vi "Periodic Tasks.vi"(8 "error in":errorcluster) -> ()   [LabVIEW 2020]
doc: "This VI runs in parallel to other robot code. It can contain as many user-defined periodic loops as you need. These can carry out PID or other sorts of timed response."
uses:
  <vilib>/Rock Robotics/WPI/Utilities/WPI_GetSetVariantRefNum.vi
  Robot Global Data.vi
  <vilib>/Rock Robotics/Network Tables/NT Write Number.vi
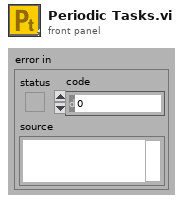
[diagram p1: front panel]
types:
  T1 = typedef "WPI_JoystickDevRef.ctl" = cluster{"Device":T2}
  T2 = typedef "WPI_JoystickDeviceEnum.ctl" = enum16{"USB 0", "USB 1", "USB 2", "USB 3", "USB 4", "USB 5"}
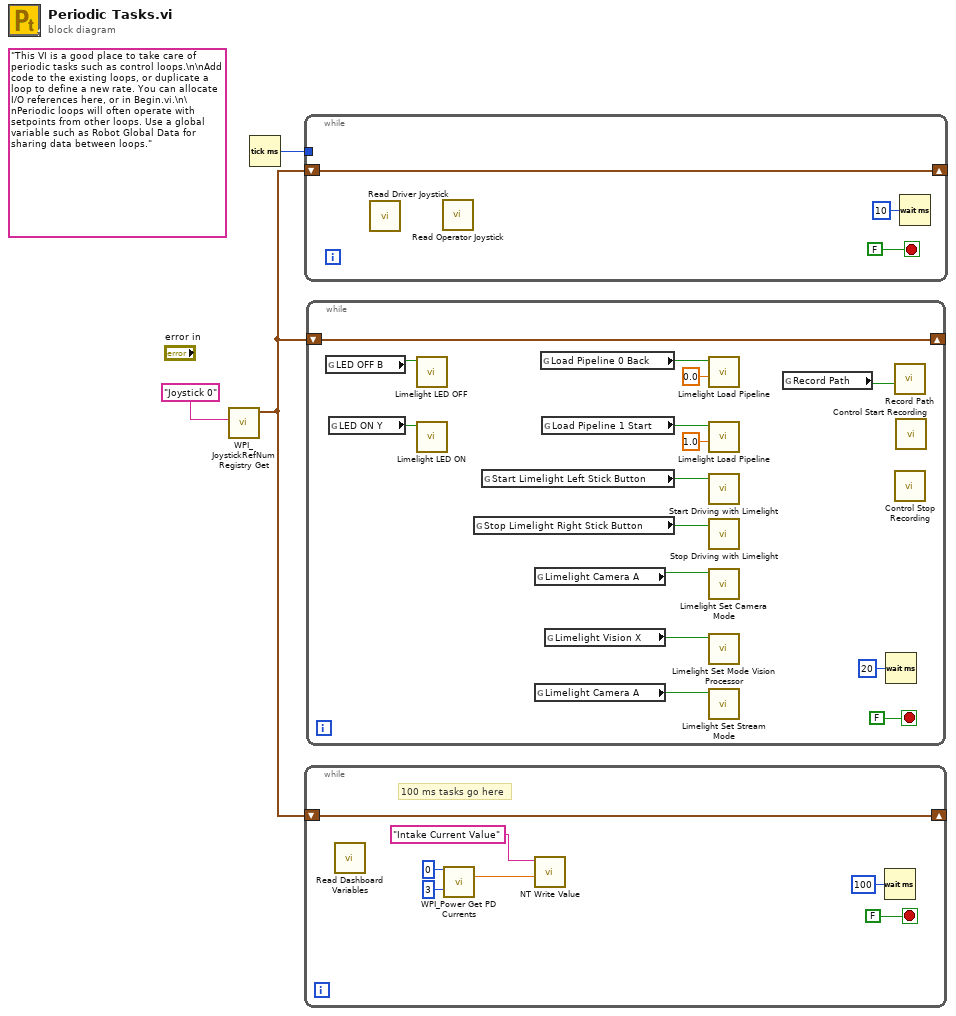
[diagram p0: block diagram]
diagram:
  (unwired) "This VI is a good place to take care of periodic tasks such as control loops.\n\nAdd code to the existing loops, or duplicate a loop to define a new rate. You can allocate I/O references here, or in Begin.vi.\n\nPeriodic loops will often operate with setpoints from other loops. Use a global variable such as Robot Global Data for sharing data between loops."
  n1 = call <vilib>:"WPI_JoystickRefNum Registry Get.vi"("refnum name"="Joystick 0") -> ("JoystickDevRef"=w1:T1)  [unwired: 1 in, 9 out]
  n2 = Tick Count (ms)() -> (millisecond timer value=w2:u32)
  n3 = while {
    shift-right: [w5] -> _
    shift-left: w1 -> [w5]
    tunnel: w2 -> [_]
    stop <- FALSE stop-if-true
    n4 = call "Read Driver Joystick.vi"() -> ()  [unwired: 12 in]
    n5 = call "Read Operator Joystick.vi"() -> ()  [unwired: 12 in]
    n6 = Wait (ms)(milliseconds to wait=u32 10) -> ()  [unwired: 1 out]
  }
  n7 = while {
    shift-right: [w11] -> _
    shift-left: w1 -> [w11]
    stop <- FALSE stop-if-true
    # "100 ms tasks go here"
    n8 = call "Read Dashboard Variables.vi"() -> ()  [unwired: 12 in]
    n9 = call <vilib>:"WPI_Power Get PD Currents.vi"("Power Distribution (def)"=u8 0, "PD Channel"=3) -> ("current (A)"=w8:dbl)  [unwired: 10 in, 3 out]
    n10 = call-poly <vilib>:"NT Write Value.vi"("Numeric"=w8, "Name"="Intake Current Value") -> ()  [unwired: 9 in, 1 out]
    n11 = Wait (ms)(milliseconds to wait=u32 100) -> ()  [unwired: 1 out]
  }
  n12 = while {
    shift-right: [w26] -> _
    shift-left: w1 -> [w26]
    stop <- FALSE stop-if-true
    n13 = global read "Robot Global Data.vi" "LED OFF B"() -> (w24:bool)
    n14 = global read "Robot Global Data.vi" "LED ON Y"() -> (w25:bool)
    n15 = call "Limelight LED OFF.vi"("D Select  8"=w24) -> ()  [unwired: 11 in]
    n16 = call "Limelight LED ON.vi"("D Start  9"=w25) -> ()  [unwired: 10 in, 1 out]
    n17 = global read "Robot Global Data.vi" "Stop Limelight Right Stick Button"() -> (w17:bool)
    n18 = global read "Robot Global Data.vi" "Start Limelight Left Stick Button"() -> (w16:bool)
    n19 = global read "Robot Global Data.vi" "Limelight Camera A"() -> (w21:bool)
    n20 = global read "Robot Global Data.vi" "Limelight Camera A"() -> (w15:bool)
    n21 = global read "Robot Global Data.vi" "Load Pipeline 0 Back"() -> (w23:bool)
    n22 = global read "Robot Global Data.vi" "Load Pipeline 1 Start"() -> (w22:bool)
    n23 = global read "Robot Global Data.vi" "Limelight Vision X"() -> (w20:bool)
    n24 = call "Limelight Load Pipeline.vi"("Pipeline Number"=0.0, "Load Pipeline"=w23) -> ()  [unwired: 10 in]
    n25 = call "Limelight Load Pipeline.vi"("Pipeline Number"=1.0, "Load Pipeline"=w22) -> ()  [unwired: 10 in]
    n26 = call "Start Driving with Limelight.vi"("Drive with Limelight"=w16) -> ()  [unwired: 11 in]
    n27 = call "Stop Driving with Limelight.vi"("Drive with Limelight"=w17) -> ()  [unwired: 11 in]
    n28 = call "Limelight Set Camera Mode.vi"("Camra"=w21) -> ()  [unwired: 11 in]
    n29 = call "Limelight Set Mode Vision Processor.vi"("Vision Processor"=w20) -> ()  [unwired: 11 in]
    n30 = call "Limelight Set Stream Mode.vi"("Camra"=w15) -> ()  [unwired: 11 in]
    n31 = global read "Robot Global Data.vi" "Record Path"() -> (w14:bool)
    n32 = Wait (ms)(milliseconds to wait=u32 20) -> ()  [unwired: 1 out]
    n33 = call "Record Path.vi"("Record Path"=w14) -> ()  [unwired: 11 in]
    n34 = call "Control Stop Recording.vi"() -> ()  [unwired: 12 in]
    n35 = call "Control Start Recording.vi"() -> ()  [unwired: 12 in]
  }
